vi "AllaxisControl.vi"() -> ()   [LabVIEW 2018]
panel:
  in  "Set target positions":bool
  in  "Stop2":bool
  out "Current Position":dbl[](array[numeric])
  out "z":dbl
  out "y":dbl
  out "x":dbl
  in  "Target Position":dbl[](array[numeric])
  out "Error Out":errorcluster
  in  "Error In":errorcluster
  out "Identification":string
  out "Axis ID´s":string[](array[string])
  out "Configuration_Setup.vi is running":bool
  in  "stop":bool
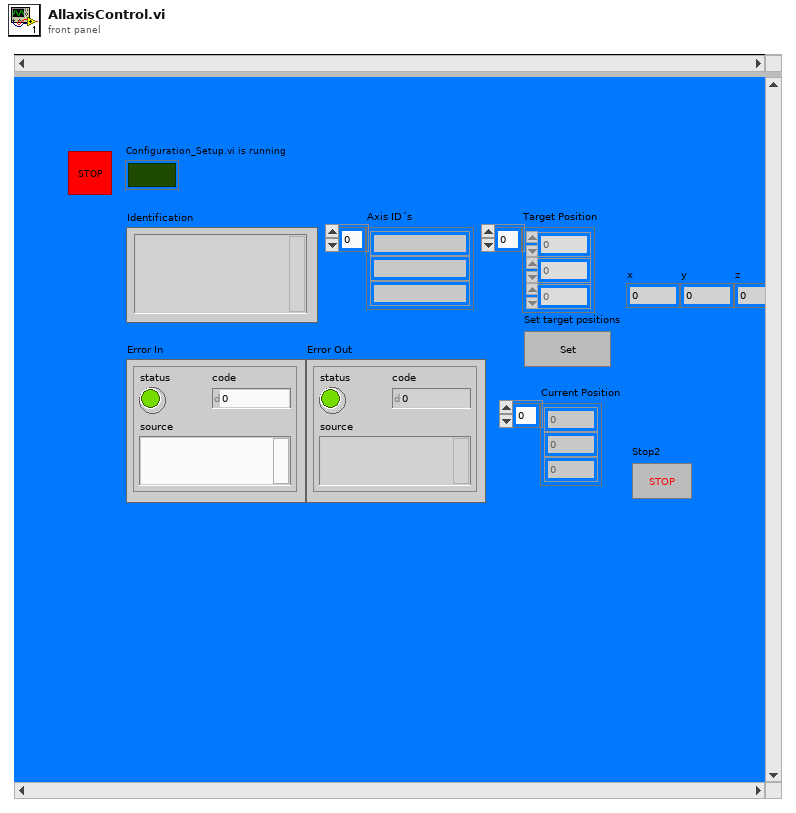
[diagram p1: front panel]
types:
  T1 = cluster{"Host address/name":string, "Port":i32, "Board":i32, "TCP/IP Search?":bool}
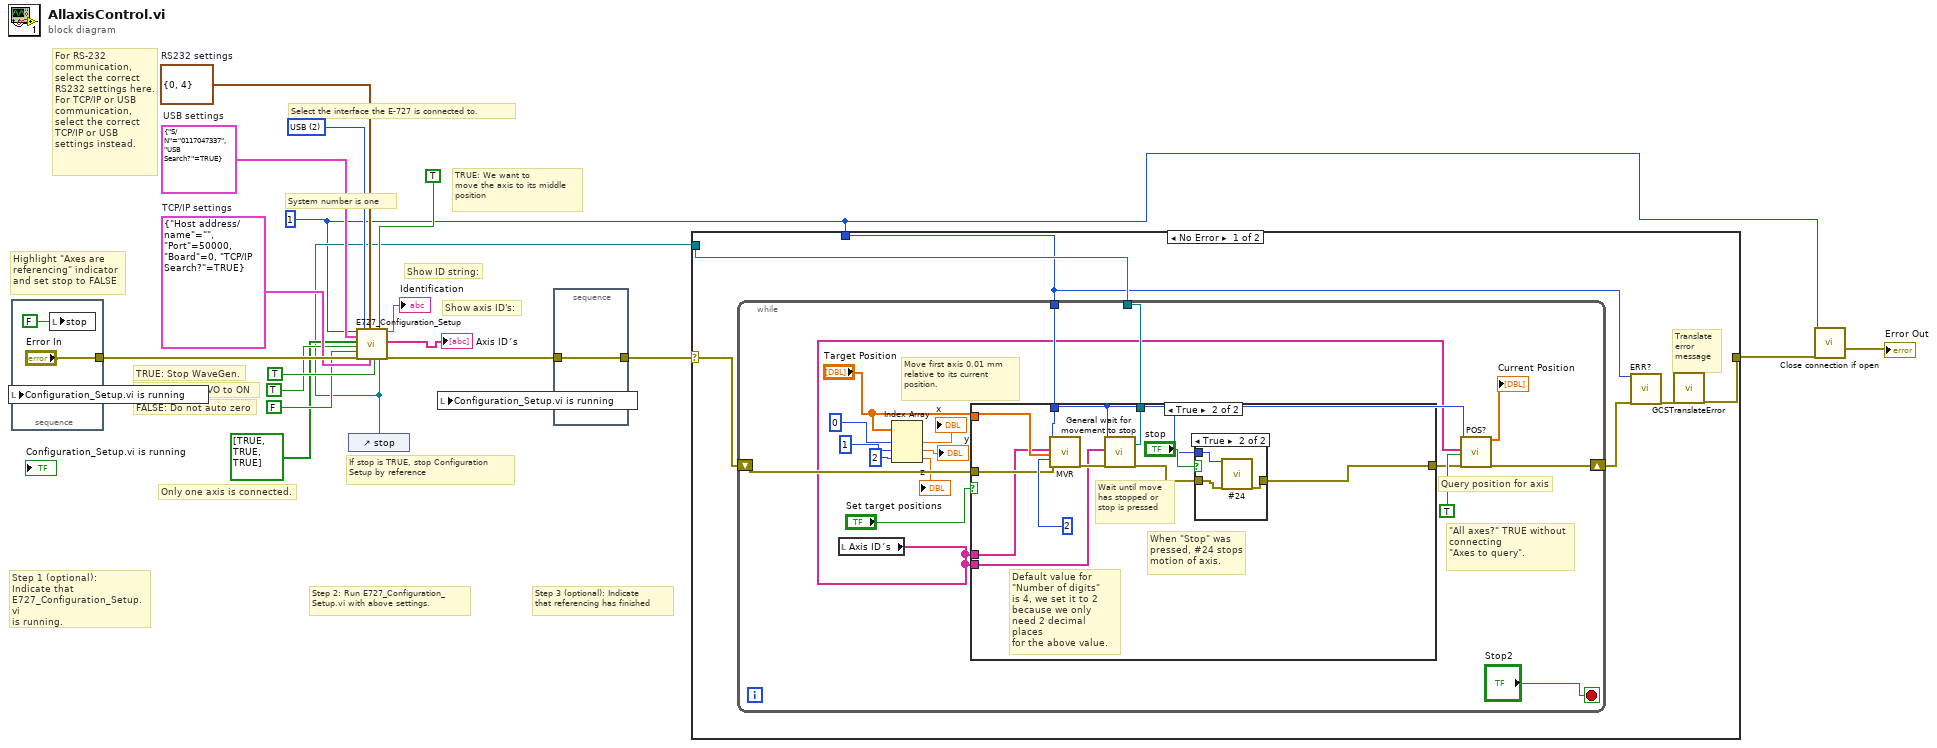
[diagram p0: block diagram]
diagram:
  w8 = cluster{"S/N":string, "USB Search?":bool} {"S/N"="0117047337", "USB Search?"=TRUE}  # USB settings
  w9 = u16 2 items=["RS232", "TCP/IP", "USB"] ("Interface")
  w11 = cluster{"Portnumber":i32, "Baudrate":u16} {"Portnumber"=0, "Baudrate"=4}  # RS232 settings
  w16 = T1 {"Host address/name"="", "Port"=50000, "Board"=0, "TCP/IP Search?"=TRUE}  # TCP/IP settings
  w5 = 1 ("System no.")
  # "Only one axis is connected."
  # "TRUE: We want to\nmove the axis to its middle\nposition"
  # "FALSE: Do not auto zero"
  # "TRUE: Switch SVO to ON"
  # "If stop is TRUE, stop Configuration\nSetup by reference"
  # "For RS-232 \ncommunication,\nselect the correct\nRS232 settings here.\nFor TCP/IP or USB \ncommunication, \nselect the correct \nTCP/IP or USB\nsettings instead."
  # "Select the interface the E-727 is connected to."
  # "Step 3 (optional): Indicate\nthat referencing has finished"
  # "Step 2: Run E727_Configuration_\nSetup.vi with above settings."
  # "Step 1 (optional): \nIndicate that\nE727_Configuration_Setup.vi\nis running."
  # "Highlight \"Axes are\nreferencing\" indicator\nand set stop to FALSE"
  # "Show axis ID's:"
  # "Show ID string:"
  # "TRUE: Stop WaveGen."
  # "System number is one"
  n1 = stacked-sequence {
    tunnel: ["Error In"] -> w17
    frame #0 {
      n2 = local write "Configuration_Setup.vi is running"(TRUE ("Configuration_Setup.vi is running")) -> ()
      n3 = local write "stop"(FALSE ("stop")) -> ()
    }
  }
  n4 = control-ref of="stop"() -> (w7:refnum<vi>)
  n5 = call "E727_Configuration_Setup.vi"("System no."=w5, "USB settings"=w8, "Are stages connected?"=bool[] [TRUE, TRUE, TRUE], "Change servo status to ON?"=TRUE ("Use dialog to define\nconnected stages?"), "Perform autozero?"=FALSE ("Use dialog to define\nconnected stages?"), "error in"=w17, "Interface"=w9, "RS232 settings"=w11, "TCP/IP settings"=w16, "Stop wave generator\noutput (if any)"=TRUE ("All axes?"), "Move to middle?"=TRUE, "Stop refnum"=w7) -> ("Identification"=→"Identification":string, "All conn. axes"=→"Axis ID´s":string[], "error out"=w18:errorcluster)  [unwired: 2 in, 3 out]
  n6 = stacked-sequence {
    tunnel: w18 -> [w23]
    tunnel: [w23] -> w4
    frame #0 {
      n7 = local write "Configuration_Setup.vi is running"(FALSE ("Configuration_Setup.vi is running")) -> ()
    }
  }
  n8 = case shown="No Error" w4 {
    selector: w4 -> [w24 w63]
    tunnel: [w29 w63] -> w6
    tunnel: w5 -> [w25 _]
    tunnel: w7 -> [w28 _]
    frame No Error {
      # "Translate\nerror \nmessage"
      n9 = while {
        tunnel: w28 -> [w45]
        tunnel: w25 -> [w42]
        shift-right: [w43] -> w27
        shift-left: w24 -> [w40]
        stop <- "Stop2" stop-if-true
        # "\"All axes?\" TRUE without connecting\n\"Axes to query\"."
        # "Move first axis 0.01 mm\nrelative to its current\nposition."
        # "Query position for axis"
        n10 = local read "Axis ID´s"() -> (w30:string[])
        n11 = Index Array(array="Target Position", index #1=0 ("index"), index #2=1 ("index"), index #3=2 ("index")) -> (element #1=→"x":dbl, element #2=→"y":dbl, element #3=→"z":dbl)
        n12 = case shown="True" "Set target positions" {
          tunnel: w45 -> [_ w56]
          tunnel: [w47 w54] -> w44
          tunnel: w42 -> [_ w52]
          tunnel: "Target Position" -> [_ w51]
          tunnel: w40 -> [w47 w50]
          tunnel: w30 -> [_ w49]
          tunnel: w30 -> [_ w48]
          frame False {
          }
          frame True {
            # "When \"Stop\" was \npressed, #24 stops\nmotion of axis."
            # "Wait until move\nhas stopped or\nstop is pressed"
            # "Default value for\n\"Number of digits\"\nis 4, we set it to 2\nbecause we only\nneed 2 decimal places\nfor the above value."
            n13 = call "MVR.vi"("System no."=w52, "Axes to move"=w48, "Position values"=w51, "No.of digits"=i16 2, "error in"=w50) -> ("error out"=w57:errorcluster)  [unwired: 14 out]
            n14 = call "General wait for movement to stop.vi"("System no."=w52, "Axes to wait for"=w49, "error in"=w57, "Stop refnum"=w56) -> ("error out"=w55:errorcluster)  [unwired: 4 in, 11 out]
            n15 = case shown="True" "stop" {
              tunnel: w55 -> [w59 w62]
              tunnel: [w59 w61] -> w54
              tunnel: w52 -> [_ w60]
              frame False {
              }
              frame True {
                n16 = call "#24.vi"("System no."=w60, "error in"=w62) -> ("error out"=w61:errorcluster)  [unwired: 17 out]
              }
            }
          }
        }
        n17 = call "POS?.vi"("System no."=w42, "Axes to query"=w30, "All axes?"=TRUE, "error in"=w44) -> ("Position"=→"Current Position":dbl[], "error out"=w43:errorcluster)  [unwired: 1 in, 13 out]
      }
      n18 = call "ERR?.vi"("System no."=w25, "error in"=w27) -> ("error out"=w26:errorcluster)  [unwired: 17 out]
      n19 = call "GCSTranslateError.vi"("error in"=w26) -> ("error out"=w29:errorcluster)  [unwired: 18 out]
    }
    frame Error {
      # "Error during initialization"
    }
  }
  n20 = call "Close connection if open.vi"("System no."=w5, "error in"=w6) -> ("error out"=→"Error Out":errorcluster)  [unwired: 1 in, 16 out]
